vi "SetExtClk.vi"(8 "error in (no error)":errorcluster, 10 "PreScale":sgl, 11 "PCA in":refnum<class "PCA.lvclass">) -> (0 "error out":errorcluster, 3 "PCA out":refnum<class "PCA.lvclass">)   [LabVIEW 2022 SP3, in "PCA9685.lvlib" / "PCA.lvclass"]
uses:
  PCA.lvclass
  PCA.lvclass/PCA.ctl
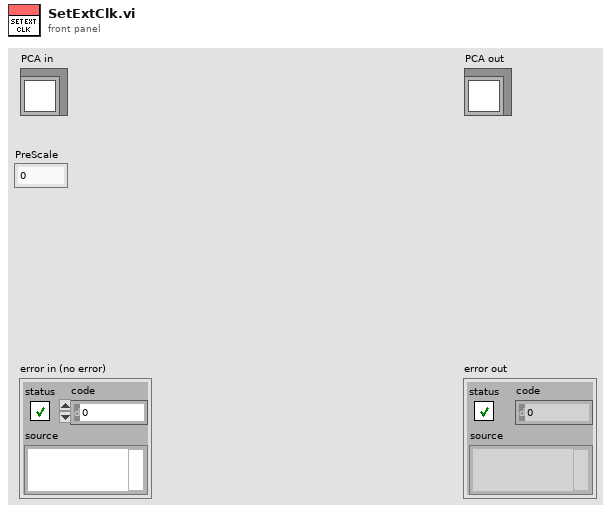
[diagram p1: front panel]
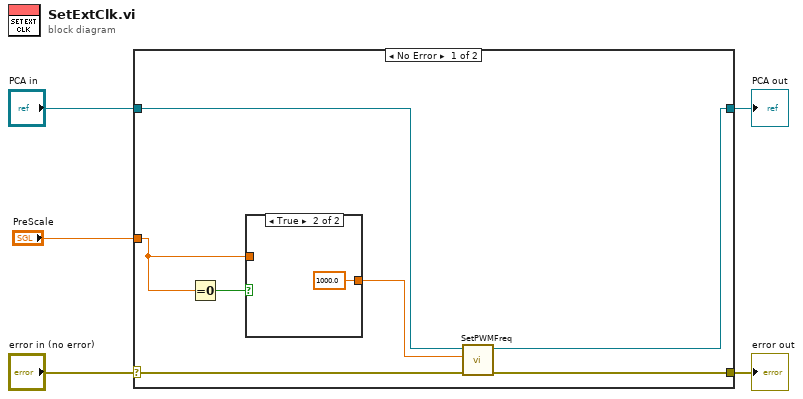
[diagram p0: block diagram]
diagram:
  n1 = case shown="No Error" "error in (no error)" {
    selector: "error in (no error)" -> [w12 w16]
    tunnel: [w11 w16] -> w4
    tunnel: [w6 w15] -> w2
    tunnel: "PCA in" -> [w10 w15]
    tunnel: "PreScale" -> [w7 _]
    frame No Error {
      n2 = Equal To 0?(x=w7) -> (x = 0?=w9:bool)
      n3 = case shown="True" w9 {
        tunnel: [w13 sgl 1000.0 ("PreScale")] -> w8
        tunnel: w7 -> [w13 _]
        frame False {
        }
        frame True {
        }
      }
      n4 = call "SetPWMFreq.vi"("error in (no error)"=w12, "Freq"=w8, "PCA in"=w10) -> ("error out"=w11:errorcluster, "PCA out"=w6:refnum<class "PCA.lvclass">)  [unwired: 7 in]
    }
    frame Error {
    }
  }
  "error out" <- w4
  "PCA out" <- w2
